vi "Wait.vi"(10 "Error in":errorcluster, 11 "Wait Time":u32) -> (7 "Error out":errorcluster)   [LabVIEW 2015]
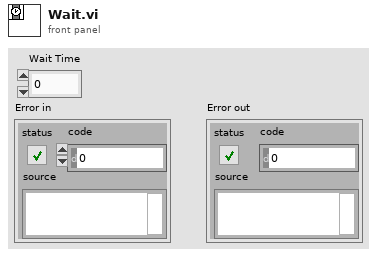
[diagram p1: front panel]
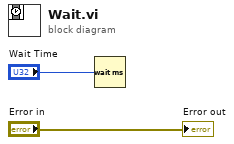
[diagram p0: block diagram]
diagram:
  n1 = Wait (ms)(milliseconds to wait="Wait Time") -> ()  [unwired: 1 out]
  "Error out" <- "Error in"
